vi "Initialize.vi"(8 "error in (no error)":errorcluster, 9 "Components":refnum<class "Component.lvclass">[](array[class]), 10 "transfer configuration":cluster{"configurations":T1[]}, 11 "Transfer Configuration in":refnum<class "Transfer Configuration.lvclass">) -> (0 "error out":errorcluster, 3 "Transfer Configuration out":refnum<class "Transfer Configuration.lvclass">)   [LabVIEW 2017, in "DSF Core.lvlib" / "Transfer Configuration.lvclass"]
uses:
  Transfer Configuration.lvclass
  Component/Component.lvclass
  Typedefs/DSF Component Configuration.ctl
  Typedefs/DSF Version Info.ctl
  Core/Channel/Core Channels Configuration.lvclass
  Transfer Configuration.lvclass/Transfer Configuration.ctl
  Configuration.lvclass
  DSF Core.lvlib
  Component Configuration/Component Configuration.lvclass
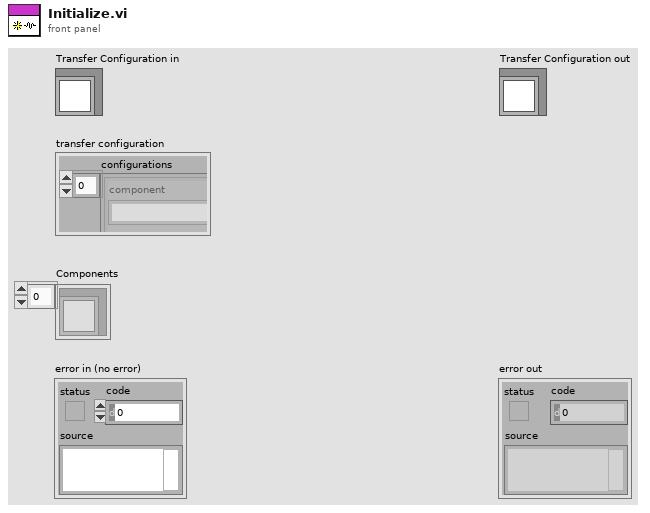
[diagram p1: front panel]
types:
  T1 = typedef "DSF Core.lvlib/DSF Component Configuration.ctl" = cluster{"component":string, "data":string, "data version":T2}
  T2 = typedef "DSF Core.lvlib/DSF Version Info.ctl" = cluster{"major":i32, "minor":i32, "fix":i32, "build":string}
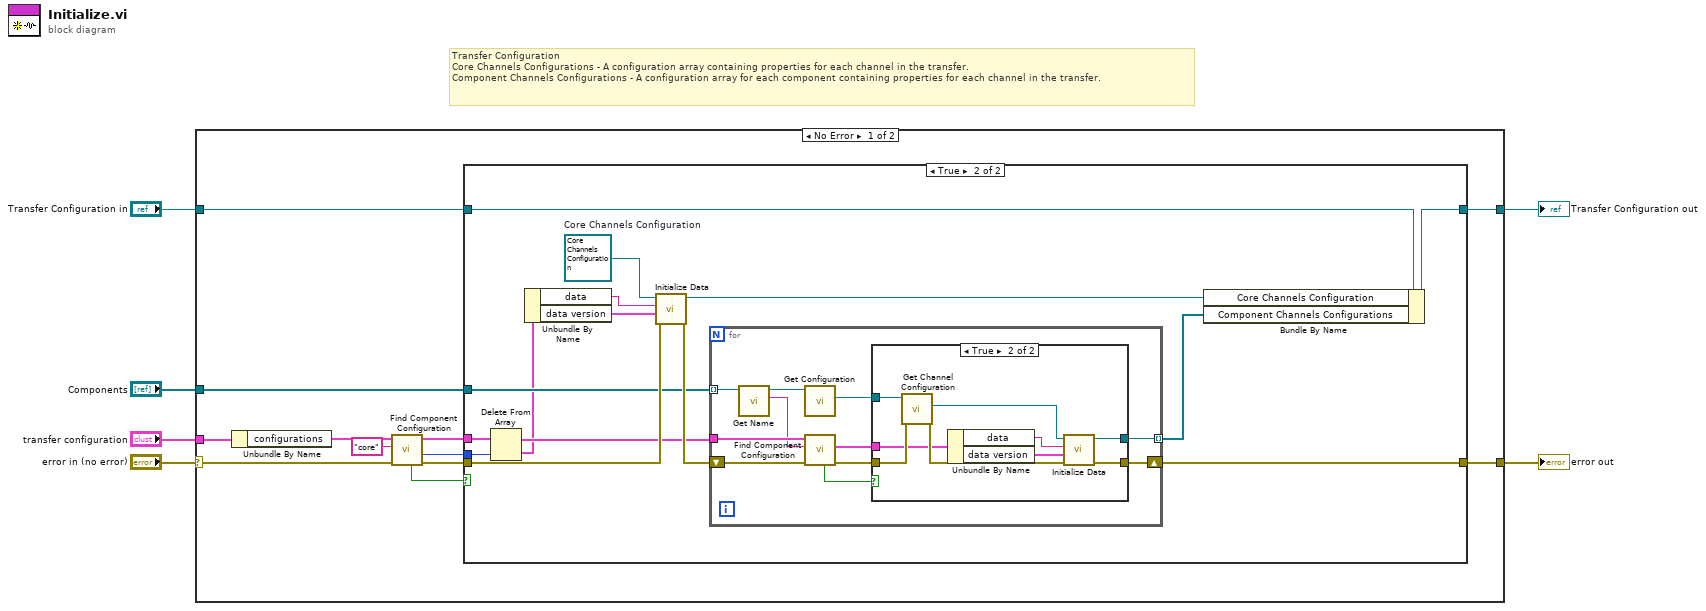
[diagram p0: block diagram]
diagram:
  # "Transfer Configuration\nCore Channels Configurations - A configuration array containing properties for each channel in the transfer.\nComponent Channels Configurations - A configuration array for each component containing properties for each channel in the transfer."
  n1 = case shown="No Error" "error in (no error)" {
    selector: "error in (no error)" -> [w7 w58]
    tunnel: "transfer configuration" -> [w18 _]
    tunnel: "Transfer Configuration in" -> [w13 w57]
    tunnel: [w12 w57] -> w4
    tunnel: "Components" -> [w9 _]
    tunnel: [w8 w58] -> w2
    frame No Error {
      n2 = Unbundle By Name(w18) -> ("configurations"=w17:T1[])
      n3 = call "Find Component Configuration.vi"("error in (no error)"=w7, "component"="core", "configurations in"=w17) -> ("error out"=w15:errorcluster, "index"=w11:i32, "configurations out"=w10:T1[], "found?"=w14:bool)  [unwired: 4 in, 1 out]
      n4 = case shown="True" w14 {
        tunnel: w15 -> [w19 w29]
        tunnel: w13 -> [w20 w31]
        tunnel: [w20 w30] -> w12
        tunnel: w11 -> [_ w27]
        tunnel: w10 -> [_ w28]
        tunnel: w9 -> [_ w24]
        tunnel: [w19 w22] -> w8
        frame False {
          # "Core configuration not found. Error."
        }
        frame True {
          w35 = refnum<class "Core Channels Configuration.lvclass"> refnum  # Core Channels Configuration
          n5 = Delete From Array(array=w28, index=w27) -> (deleted portion=w21:T1, array with subset deleted=w25:T1[])  [unwired: 1 in]
          n6 = Unbundle By Name(w21) -> ("data"=w33:string, "data version"=w34:T2)
          n7 = call-dynamic "Initialize Data.vi"("error in (no error)"=w29, "data version"=w34, "data"=w33, "Core Channel Configuration in"=w35) -> ("error out"=w26:errorcluster, "Core Channel Configuration out"=w32:refnum<class "Core Channels Configuration.lvclass">)  [unwired: 6 in]
          n8 = for {
            tunnel: w24 -> [w40] mode=indexing
            tunnel: w25 -> [w42]
            shift-right: [w44] -> w22
            shift-left: w26 -> [w38]
            tunnel: [w41] -> w23 mode=indexing
            n9 = call "Get Name.vi"("Component in"=w40) -> ("name"=w39:string, "Component out"=w37:refnum<class "Component.lvclass">)  [unwired: 9 in]
            n10 = call "Get Configuration.vi"("Component in"=w37) -> ("Configuration"=w36:refnum<class "Component Configuration.lvclass">)  [unwired: 9 in, 1 out]
            n11 = call "Find Component Configuration.vi"("error in (no error)"=w38, "component"=w39, "configurations in"=w42) -> ("error out"=w45:errorcluster, "component configuration"=w43:T1, "found?"=w46:bool)  [unwired: 4 in, 2 out]
            n12 = case shown="True" w46 {
              tunnel: w45 -> [w47 w56]
              tunnel: [w47 w55] -> w44
              tunnel: w43 -> [_ w52]
              tunnel: [_ w49] -> w41
              tunnel: w36 -> [_ w48]
              frame False {
              }
              frame True {
                n13 = call "Get Channel Configuration.vi"("error in (no error)"=w56, "Component Configuration in"=w48) -> ("error out"=w54:errorcluster, "Channel Configuration"=w53:refnum<class "Configuration.lvclass">)  [unwired: 7 in, 1 out]
                n14 = Unbundle By Name(w52) -> ("data"=w51:string, "data version"=w50:T2)
                n15 = call-dynamic "Initialize Data.vi"("error in (no error)"=w54, "data version"=w50, "data"=w51, "Configuration in"=w53) -> ("error out"=w55:errorcluster, "Configuration out"=w49:refnum<class "Configuration.lvclass">)  [unwired: 6 in]
              }
            }
          }
          n16 = Bundle By Name(cluster=w31, "Core Channels Configuration"=w32, "Component Channels Configurations"=w23) -> (w30:refnum<class "Transfer Configuration.lvclass">)
        }
      }
    }
    frame Error {
    }
  }
  "error out" <- w2
  "Transfer Configuration out" <- w4
